vi "Main.vi"(11 "Module Admin":refnum<class "Delacor_lib_QMH_Cloneable Module Admin.lvclass">) -> ()   [LabVIEW 2023, in "EL72xx_DMC_ServoAxis.lvlib"]
doc: "This template is based off of the Queued Message Handler design pattern and the Queued Message Handler project template that ships with LabVIEW.\n\nThe main difference is that the queue is private to this module and communication between modules is performed via Broadcast and Request events.\n\nRequest events are wrapped in public API methods and are handled in the Event Handling Loop (EHL) of this VI. Any module can register for Broadcast events sent by this module. The EHL generates messages based on user interface actions.\n\nThe Message Handling Loop (MHL) processes messages generated by the EHL, or by other messages. The messages are string values, so new messages can be added easily to the Message Cases case structure in the MHL. Each message cluster can also provide an optional value for Message Data, which is a variant that can be converted to whatever message-specific data is required.\n_____\nBased on DQMH Project Template 7.0.1.1316."
uses:
  EL72xx_DMC_ServoAxis.lvlib
  <vilib>/Delacor/Delacor QMH/Libraries/Cloneable Module Admin_class/Delacor_lib_QMH_Cloneable Module Admin.lvclass
  C:/Program Files/National Instruments/LabVIEW 2023/vi.lib/Delacor/Delacor QMH/Libraries/Module Admin_class/Delacor_lib_QMH_Module Admin.lvclass
  Module Data--cluster.ctl
  <vilib>/Delacor/Delacor QMH/Libraries/Message Queue_class/Delacor_lib_QMH_Message Queue.lvclass/Delacor_lib_QMH_Message Queue.ctl
  <vilib>/Delacor/Delacor QMH/Libraries/Cloneable Module Admin_class/Delacor_lib_QMH_Cloneable Module Admin.lvclass/Delacor_lib_QMH_Cloneable Module Admin.ctl
  Stop Argument--cluster.ctl
  <vilib>/Delacor/Delacor QMH/Libraries/Module Admin_class/Delacor_lib_QMH_Module Admin.lvclass/Delacor_lib_QMH_Module Admin.ctl
  Enable_Drive Argument--cluster.ctl
  <vilib>/Utility/miscctls.llb/LVPointTypeDef.ctl
  <vilib>/Delacor/Delacor QMH/Libraries/Message Queue_class/Delacor_lib_QMH_Enqueue Message (Single).vi
  <vilib>/Delacor/Delacor QMH/Libraries/Cloneable Module Admin_class/Delacor_lib_QMH_Get Module ID.vi
  <vilib>/Delacor/Delacor QMH/Libraries/Module Admin_class/Delacor_lib_QMH_Get External Launch.vi
  <vilib>/Delacor/Delacor QMH/Libraries/Message Queue_class/Delacor_lib_QMH_Message Queue.lvclass
  ConnectToDrive Argument--cluster.ctl
  DisconnectFromDrive Argument--cluster.ctl
  DisableDrive Argument--cluster.ctl
  <userlib>/Beckhoff-LabVIEW-Interface/_DependsOn/Base/TypeResolver/Set TypeResolver.vi
  <userlib>/Beckhoff-LabVIEW-Interface/_DependsOn/Base/Write/Write Sync.vi
panel:
  out "error out":errorcluster
  out "Status":string
  in  "Simulate EHL Error":bool
  in  "Simulate MHL Error":bool
  # "Other processes communicate with this Module via its Public API (wrappers for its Request Events).\n\nThis Module communicates with other processes via its Broadcast Events.\nAny process that wants to receive these messages can register for this module's Broadcast events."
  # "This template is for the DQMH framework. See the block diagram for more information on how to use this template."
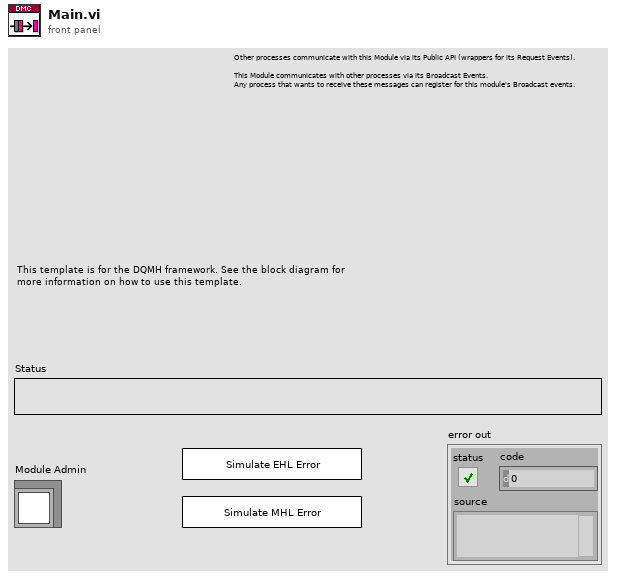
[diagram p1: front panel]
types:
  T1 = typedef "EL72xx_DMC_ServoAxis.lvlib/Request Events--cluster.ctl" = cluster{"Stop Module":refnum<user-event>, "Show Panel":refnum<user-event>, "Hide Panel":refnum<user-event>, "Show Diagram":refnum<user-event>, "Get Module Execution Status":refnum<user-event>, "Enable_Drive":refnum<user-event>, "ConnectToDrive":refnum<user-event>, "DisconnectFromDrive":refnum<user-event>, "DisableDrive":refnum<user-event>}
  T2 = typedef "EL72xx_DMC_ServoAxis.lvlib/Module Data--cluster.ctl" = cluster{"Status":string}
  T3 = enum32{"invalid lock state", "Not Locked", "Locked (No Password)", "Password-protected"}
  T4 = typedef "EL72xx_DMC_ServoAxis.lvlib/Stop Argument--cluster.ctl" = cluster{"Module ID":i32, "Origin":string, "Exit via Stop Module Req?":bool, "Wait for Module to stop?":bool}
  T5 = typedef "EL72xx_DMC_ServoAxis.lvlib/Enable_Drive Argument--cluster.ctl" = cluster{"Module ID":i32, "Enable":bool}
  T6 = typedef "EL72xx_DMC_ServoAxis.lvlib/ConnectToDrive Argument--cluster.ctl" = cluster{"Module ID":i32, "Path":path}
  T7 = typedef "EL72xx_DMC_ServoAxis.lvlib/DisconnectFromDrive Argument--cluster.ctl" = cluster{"Module ID":i32, "Boolean":bool}
  T8 = typedef "EL72xx_DMC_ServoAxis.lvlib/DisableDrive Argument--cluster.ctl" = cluster{"Module ID":i32, "Disable":bool}
  T9 = typedef "LVPointTypeDef.ctl" = cluster{"Horizontal":i16, "Vertical":i16}
  T10 = enum32{"Invalid", "Standard", "Closed", "Hidden", "Minimized", "Maximized"}
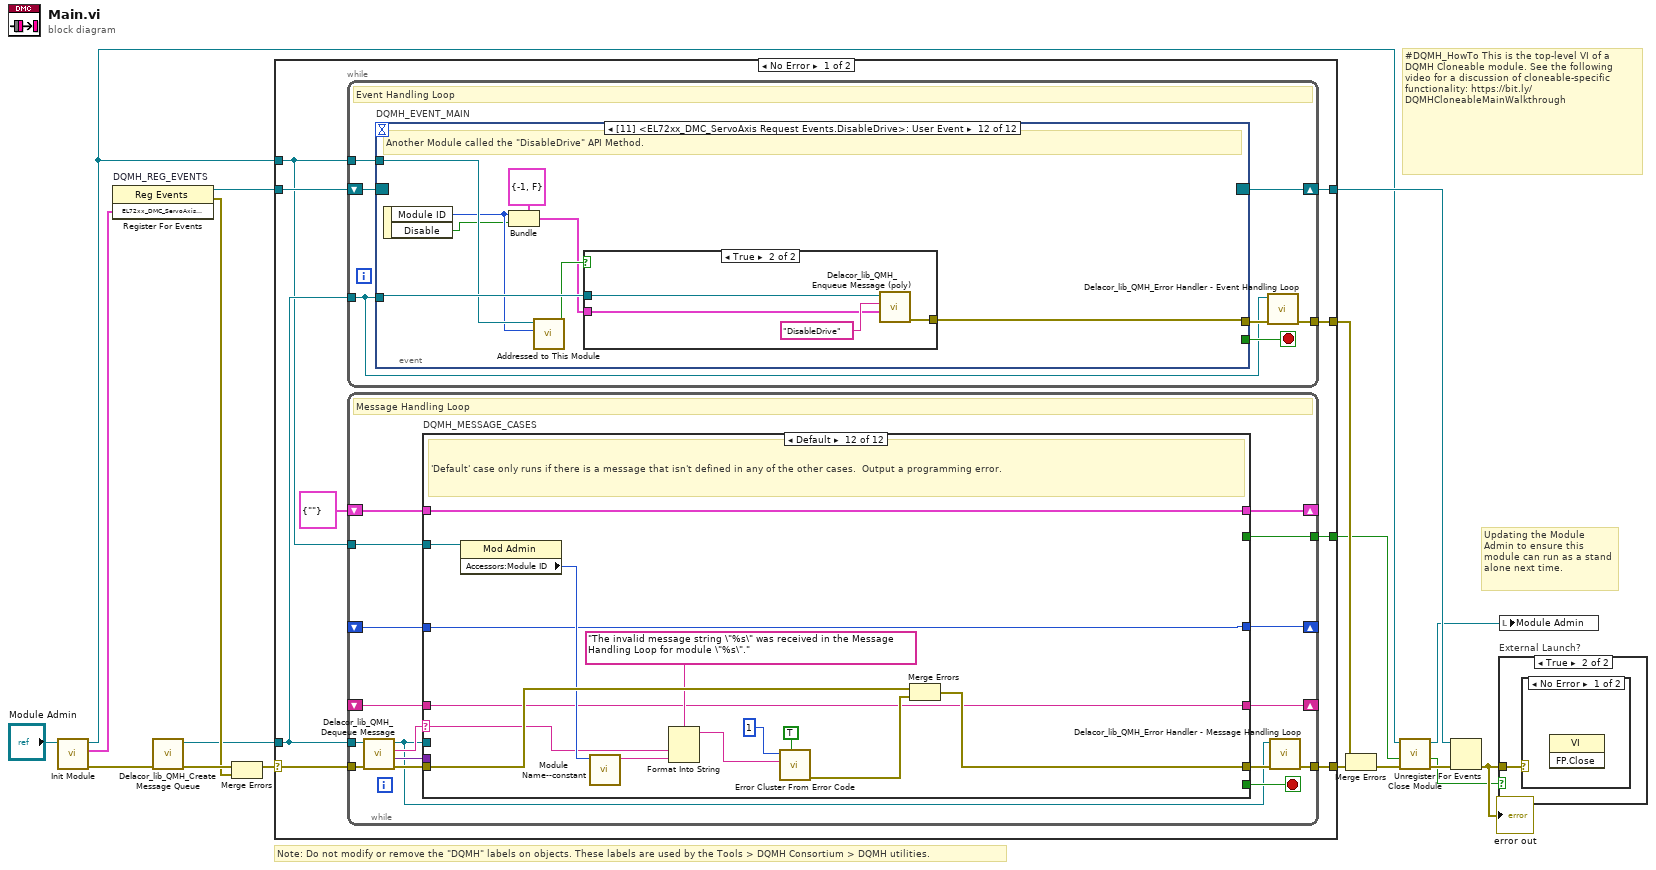
[diagram p0: block diagram]
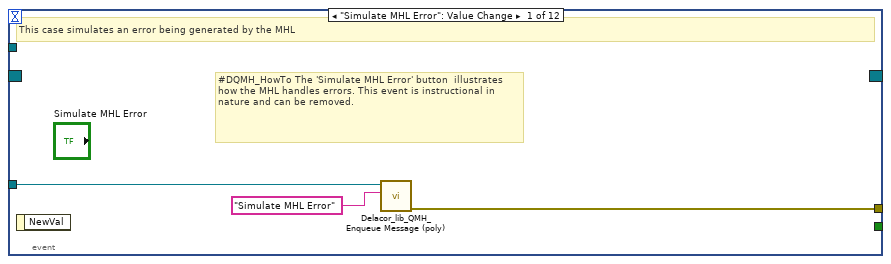
[diagram p2: hidden frame]
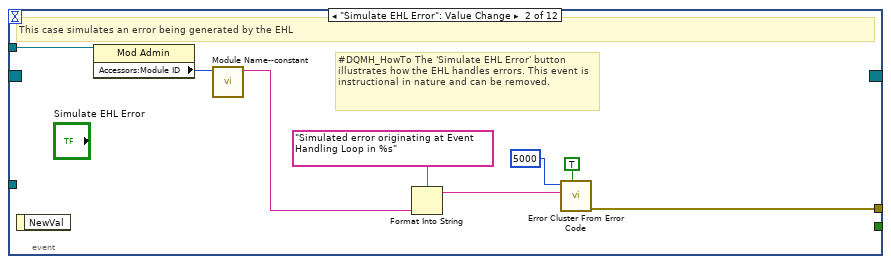
[diagram p3: hidden frame]
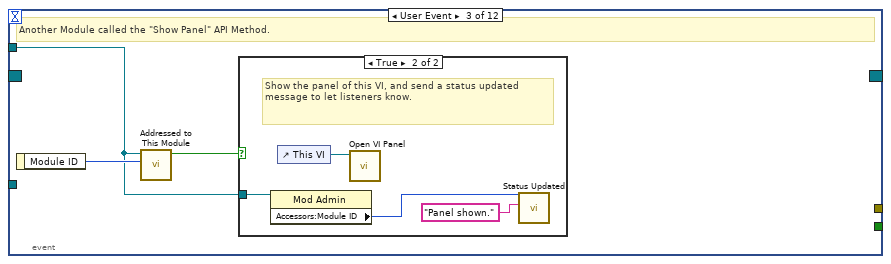
[diagram p4: hidden frame]
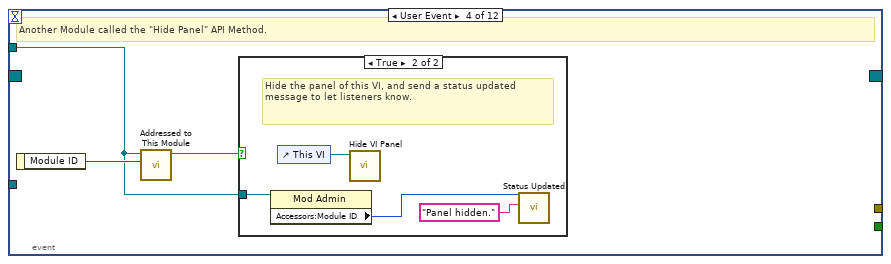
[diagram p6: hidden frame]
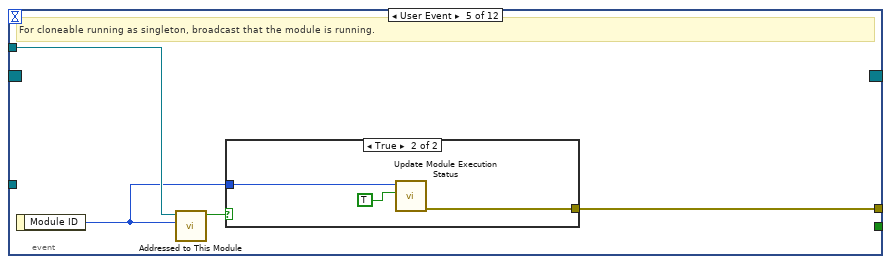
[diagram p8: hidden frame]
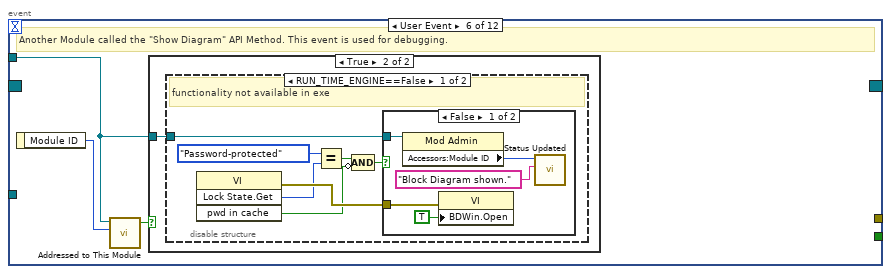
[diagram p10: hidden frame]
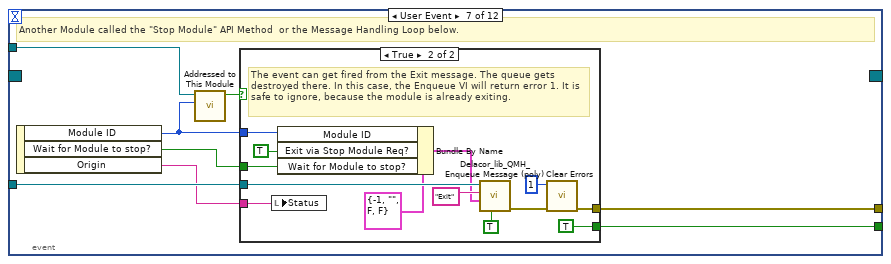
[diagram p14: hidden frame]
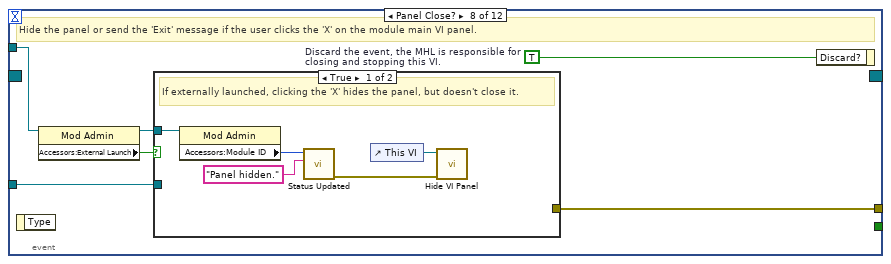
[diagram p16: hidden frame]
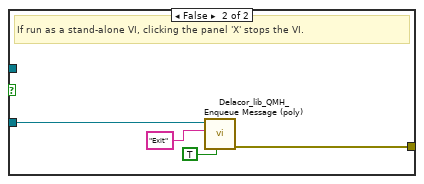
[diagram p17: hidden frame]
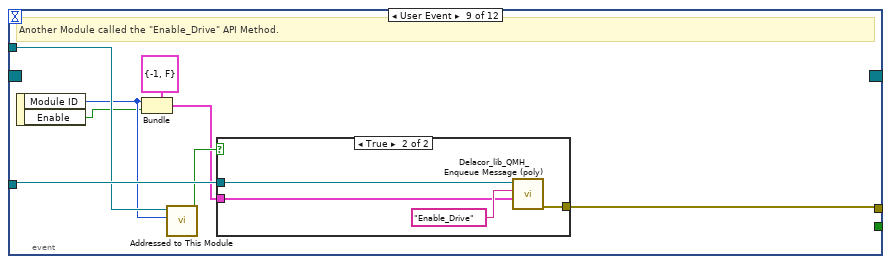
[diagram p18: hidden frame]
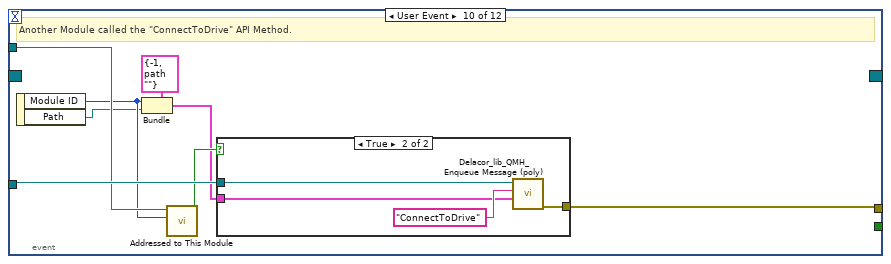
[diagram p20: hidden frame]
diagram:
  # "#DQMH_HowTo This is the top-level VI of a DQMH Cloneable module. See the following video for a discussion of cloneable-specific functionality: https://bit.ly/DQMHCloneableMainWalkthrough"
  # "Note: Do not modify or remove the \"DQMH\" labels on objects. These labels are used by the Tools > DQMH Consortium > DQMH utilities."
  # "Updating the Module Admin to ensure this module can run as a stand alone next time."
  n1 = call "Init Module.vi"("Cloneable Module Admin in"="Module Admin") -> ("error out"=w15:errorcluster, "EL72xx_DMC_ServoAxis Request Events"=w7:T1, "Cloneable Module Admin out"=w4:refnum<class "Delacor_lib_QMH_Cloneable Module Admin.lvclass">)  [unwired: 8 in]
  n2 = register-events "DQMH_REG_EVENTS"(w7) -> (reference out=w8:refnum<event-registration>, error out=w10:errorcluster)  [unwired: 2 in]
  n3 = call <vilib>:"Delacor_lib_QMH_Create Message Queue.vi"("error in"=w15) -> ("error out"=w12:errorcluster, "Message Queue"=w6:refnum<class "Delacor_lib_QMH_Message Queue.lvclass">)  [unwired: 9 in]
  n4 = Merge Errors(w12, w10) -> (w11:errorcluster)
  n5 = case shown="No Error" w11 {
    selector: w11 -> [w25 w348]
    tunnel: [w27 w347] -> w16
    tunnel: [w24 w346] -> w9
    tunnel: w8 -> [w22 w346]
    tunnel: w6 -> [w21 w339]
    tunnel: [w26 _] -> w17
    tunnel: w4 -> [w20 w342]
    tunnel: [w19 _] -> w2
    frame No Error {
      n6 = while {
        tunnel: w21 -> [w28]
        shift-right: [w31] -> w24
        shift-left: w22 -> [w32]
        tunnel: [w33] -> w26
        tunnel: w20 -> [w29]
        stop <- w30 stop-if-true
        # "Event Handling Loop"
        n7 = event "DQMH_EVENT_MAIN" shown="[11] <EL72xx_DMC_ServoAxis Request Events.DisableDrive>: User Event" {
          selector: w32 -> [_ _ _ _ _ _ _ _ _ _ _ _]
          dyn-events: [_ _ _ _ _ _ _ _ _ _ _ _] -> w31
          timeout: _ -> [_ _ _ _ _ _ _ _ _ _ _ _]
          tunnel: [_ _ _ _ _ _ w86 _ _ _ _ _] -> w30
          tunnel: w28 -> [w36 _ _ _ _ _ w89 w106 w126 w138 w150 w162]
          tunnel: [w37 w45 _ _ w63 _ w90 w109 w119 w131 w143 w155] -> w34
          tunnel: w29 -> [_ w44 w46 w53 w61 w67 w88 w107 w124 w136 w148 w160]
          event "Simulate MHL Error": Value Change {
            # "#DQMH_HowTo The 'Simulate MHL Error' button  illustrates how the MHL handles errors. This event is instructional in nature and can be removed."
            # "This case simulates an error being generated by the MHL"
            n8 = event-data() -> ()  [unwired: 1 in, 1 out]
            n9 = call-poly <vilib>:"Delacor_lib_QMH_Enqueue Message (poly).vi"("Message"="Simulate MHL Error", "Message Queue in"=w36) -> ("error out"=w37:errorcluster)  [unwired: 8 in, 1 out]
          }
          event "Simulate EHL Error": Value Change {
            # "#DQMH_HowTo The 'Simulate EHL Error' button  illustrates how the EHL handles errors. This event is instructional in nature and can be removed."
            # "This case simulates an error being generated by the EHL"
            n10 = event-data() -> ()  [unwired: 1 in, 1 out]
            n11 = property on="Property Node" class="Mod Admin"(reference=w44) -> ("Accessors:Module ID"=w43:i32)  [unwired: 1 in, 2 out]
            n12 = call "Module Name--constant.vi"("Module ID"=w43) -> ("Module Name"=w38:string)  [unwired: 10 in]
            n13 = Format Into String(format string="Simulated error originating at Event Handling Loop in %s", w38) -> (resulting string=w41:string)  [unwired: 2 in, 1 out]
            n14 = call <vilib>:"Error Cluster From Error Code.vi"("show call chain? (False)"=TRUE, "error message (\"\")"=w41, "error code (0)"=5000) -> ("error out"=w45:errorcluster)  [unwired: 6 in]
          }
          event User Event {
            # "Another Module called the \"Show Panel\" API Method."
            n15 = event-data() -> ("Module ID"=w47:i32)  [unwired: 1 in]
            n16 = call "Addressed to This Module.vi"("Module ID from Argument"=w47, "Module Admin"=w46) -> ("Addressed to this instance?"=w48:bool)  [unwired: 8 in, 1 out]
            n17 = case shown="True" w48 {
              tunnel: w46 -> [_ w50]
              frame False {
              }
              frame True {
                # "Show the panel of this VI, and send a status updated message to let listeners know."
                n18 = property on="Property Node" class="Mod Admin"(reference=w50) -> ("Accessors:Module ID"=w49:i32)  [unwired: 1 in, 2 out]
                n19 = control-ref of="This VI"() -> (w52:refnum<vi>)
                n20 = call "Open VI Panel.vi"("VI"=w52) -> ()  [unwired: 10 in, 1 out]
                n21 = call "Status Updated.vi"("Status"="Panel shown." ("format string"), "Module ID"=w49) -> ()  [unwired: 9 in, 1 out]
              }
            }
          }
          event User Event {
            # "Another Module called the \"Hide Panel\" API Method."
            n22 = event-data() -> ("Module ID"=w54:i32)  [unwired: 1 in]
            n23 = call "Addressed to This Module.vi"("Module ID from Argument"=w54, "Module Admin"=w53) -> ("Addressed to this instance?"=w55:bool)  [unwired: 8 in, 1 out]
            n24 = case shown="True" w55 {
              tunnel: w53 -> [_ w57]
              frame False {
              }
              frame True {
                # "Hide the panel of this VI, and send a status updated message to let listeners know."
                n25 = property on="Property Node" class="Mod Admin"(reference=w57) -> ("Accessors:Module ID"=w56:i32)  [unwired: 1 in, 2 out]
                n26 = control-ref of="This VI"() -> (w59:refnum<vi>)
                n27 = call "Hide VI Panel.vi"("VI"=w59) -> ()  [unwired: 10 in, 1 out]
                n28 = call "Status Updated.vi"("Status"="Panel hidden." ("format string"), "Module ID"=w56) -> ()  [unwired: 9 in, 1 out]
              }
            }
          }
          event User Event {
            # "For cloneable running as singleton, broadcast that the module is running."
            n29 = event-data() -> ("Module ID"=w60:i32)  [unwired: 1 in]
            n30 = call "Addressed to This Module.vi"("Module ID from Argument"=w60, "Module Admin"=w61) -> ("Addressed to this instance?"=w62:bool)  [unwired: 8 in, 1 out]
            n31 = case shown="True" w62 {
              tunnel: [_ w66] -> w63
              tunnel: w60 -> [_ w65]
              frame False {
              }
              frame True {
                n32 = call "Update Module Execution Status.vi"("Running?"=TRUE, "Module ID"=w65) -> ("error out"=w66:errorcluster)  [unwired: 9 in]
              }
            }
          }
          event User Event {
            # "Another Module called the \"Show Diagram\" API Method. This event is used for debugging."
            n33 = event-data() -> ("Module ID"=w68:i32)  [unwired: 1 in]
            n34 = call "Addressed to This Module.vi"("Module ID from Argument"=w68, "Module Admin"=w67) -> ("Addressed to this instance?"=w69:bool)  [unwired: 8 in, 1 out]
            n35 = case shown="True" w69 {
              tunnel: w67 -> [_ w70]
              frame False {
              }
              frame True {
                n36 = disable-structure shown="RUN_TIME_ENGINE==False" {
                  disable-tunnel: w70 -> [w71 _]
                  frame condition #0 (active) {
                    # "functionality not available in exe"
                    n37 = invoke on="Invoke Node" class="VI" method="Lock State.Get"() -> (error out=w77:errorcluster, "Get Lock State"=w76:T3, "pwd in cache"=w73:bool)  [unwired: 4 in, 1 out]
                    n38 = Equal?(x=T3."Password-protected", y=w76) -> (x = y?=w74:bool)
                    n39 = Compound Arithmetic op=AND(w74, invert w73) -> (w72:bool)
                    n40 = case shown="False" w72 {
                      tunnel: w77 -> [w82 _]
                      tunnel: w71 -> [w79 _]
                      frame False {
                        n41 = property on="Property Node" class="Mod Admin"(reference=w79) -> ("Accessors:Module ID"=w78:i32)  [unwired: 1 in, 2 out]
                        n42 = property on="Property Node" class="VI"(error in=w82, "BDWin.Open"=TRUE ("Block Diagram Window:Open")) -> ()  [unwired: 1 in, 2 out]
                        n43 = call "Status Updated.vi"("Status"="Block Diagram shown." ("format string"), "Module ID"=w78) -> ()  [unwired: 9 in, 1 out]
                      }
                      frame True {
                        # "Password-protected VI, and the password is not in the cache. Do not show the diagram."
                      }
                    }
                  }
                  frame condition #1 {
                  }
                }
              }
            }
          }
          event User Event {
            # "Another Module called the \"Stop Module\" API Method  or the Message Handling Loop below."
            n44 = event-data() -> ("Module ID"=w84:i32, "Wait for Module to stop?"=w85:bool, "Origin"=w83:string)  [unwired: 1 in]
            n45 = call "Addressed to This Module.vi"("Module ID from Argument"=w84, "Module Admin"=w88) -> ("Addressed to this instance?"=w87:bool)  [unwired: 8 in, 1 out]
            n46 = case shown="True" w87 {
              tunnel: [_ w102] -> w90
              tunnel: w89 -> [_ w98]
              tunnel: [_ TRUE] -> w86
              tunnel: w85 -> [_ w93]
              tunnel: w84 -> [_ w95]
              tunnel: w83 -> [_ w91]
              frame False {
              }
              frame True {
                # "The event can get fired from the Exit message. The queue gets destroyed there. In this case, the Enqueue VI will return error 1. It is safe to ignore, because the module is already exiting."
                n47 = local write "Status"(w91) -> ()
                n48 = Bundle By Name(cluster=T4 {"Module ID"=-1, "Origin"="", "Exit via Stop Module Req?"=FALSE, "Wait for Module to stop?"=FALSE} ("Stop Argument"), "Module ID"=w95, "Exit via Stop Module Req?"=TRUE, "Wait for Module to stop?"=w93) -> (w92:T4)
                n49 = call-poly <vilib>:"Delacor_lib_QMH_Enqueue Message (poly).vi"("Priority Message? (F)"=TRUE, "Message Data"=w92, "Message"="Exit", "Message Queue in"=w98) -> ("error out"=w103:errorcluster)  [unwired: 6 in, 1 out]
                n50 = call <vilib>:"Clear Errors.vi"("error in (no error)"=w103, "specific error code to clear (0: all)"=1) -> ("error out"=w102:errorcluster)  [unwired: 4 in, 1 out]
              }
            }
          }
          event Panel Close? {
            w108 = TRUE  # Discard the event, the MHL is responsible for closing and stopping this VI.
            # "Hide the panel or send the 'Exit' message if the user clicks the 'X' on the module main VI panel."
            n51 = event-data() -> ()  [unwired: 1 in, 1 out]
            n52 = property on="Property Node" class="Mod Admin"(reference=w107) -> (reference out=w104:refnum<class "Delacor_lib_QMH_Cloneable Module Admin.lvclass">, "Accessors:External Launch"=w105:bool)  [unwired: 1 in, 1 out]
            n53 = case shown="True" w105 {
              tunnel: w106 -> [_ w117]
              tunnel: [_ w118] -> w109
              tunnel: w104 -> [w112 _]
              frame True {
                # "If externally launched, clicking the 'X' hides the panel, but doesn't close it."
                n54 = property on="Property Node" class="Mod Admin"(reference=w112) -> ("Accessors:Module ID"=w111:i32)  [unwired: 1 in, 2 out]
                n55 = call "Status Updated.vi"("Status"="Panel hidden." ("format string"), "Module ID"=w111) -> ("error out"=w110:errorcluster)  [unwired: 9 in]
                n56 = control-ref of="This VI"() -> (w114:refnum<vi>)
                n57 = call "Hide VI Panel.vi"("error in"=w110, "VI"=w114) -> ()  [unwired: 9 in, 1 out]
              }
              frame False {
                # "If run as a stand-alone VI, clicking the panel 'X' stops the VI."
                n58 = call-poly <vilib>:"Delacor_lib_QMH_Enqueue Message (poly).vi"("Priority Message? (F)"=TRUE, "Message"="Exit", "Message Queue in"=w117) -> ("error out"=w118:errorcluster)  [unwired: 7 in, 1 out]
              }
            }
            n59 = event-data ("Event Filter Node")("Discard?"=w108) -> ()  [unwired: 1 in, 1 out]
          }
          event User Event {
            # "Another Module called the \"Enable_Drive\" API Method."
            n60 = event-data() -> ("Module ID"=w121:i32, "Enable"=w120:bool)  [unwired: 1 in]
            n61 = Bundle(cluster=T5 {"Module ID"=-1, "Enable"=FALSE} ("Enable_Drive Argument"), "Module ID"=w121, "Enable"=w120) -> (w122:T5)
            n62 = call "Addressed to This Module.vi"("Module ID from Argument"=w121, "Module Admin"=w124) -> ("Addressed to this instance?"=w125:bool)  [unwired: 8 in, 1 out]
            n63 = case shown="True" w125 {
              tunnel: w126 -> [_ w130]
              tunnel: w122 -> [_ w128]
              tunnel: [_ w127] -> w119
              frame False {
              }
              frame True {
                n64 = call-poly <vilib>:"Delacor_lib_QMH_Enqueue Message (poly).vi"("Message Data"=w128, "Message"="Enable_Drive", "Message Queue in"=w130) -> ("error out"=w127:errorcluster)  [unwired: 7 in, 1 out]
              }
            }
          }
          event User Event {
            # "Another Module called the \"ConnectToDrive\" API Method."
            n65 = event-data() -> ("Module ID"=w133:i32, "Path"=w132:path)  [unwired: 1 in]
            n66 = Bundle(cluster=T6 {"Module ID"=-1, "Path"=path ""} ("ConnectToDrive Argument"), "Module ID"=w133, "Path"=w132) -> (w134:T6)
            n67 = call "Addressed to This Module.vi"("Module ID from Argument"=w133, "Module Admin"=w136) -> ("Addressed to this instance?"=w137:bool)  [unwired: 8 in, 1 out]
            n68 = case shown="True" w137 {
              tunnel: w138 -> [_ w142]
              tunnel: w134 -> [_ w140]
              tunnel: [_ w139] -> w131
              frame False {
              }
              frame True {
                n69 = call-poly <vilib>:"Delacor_lib_QMH_Enqueue Message (poly).vi"("Message Data"=w140, "Message"="ConnectToDrive", "Message Queue in"=w142) -> ("error out"=w139:errorcluster)  [unwired: 7 in, 1 out]
              }
            }
          }
          event User Event {
            # "Another Module called the \"DisconnectFromDrive\" API Method."
            n70 = event-data() -> ("Module ID"=w145:i32, "Boolean"=w144:bool)  [unwired: 1 in]
            n71 = Bundle(cluster=T7 {"Module ID"=-1, "Boolean"=FALSE} ("DisconnectFromDrive Argument"), "Module ID"=w145, "Boolean"=w144) -> (w146:T7)
            n72 = call "Addressed to This Module.vi"("Module ID from Argument"=w145, "Module Admin"=w148) -> ("Addressed to this instance?"=w149:bool)  [unwired: 8 in, 1 out]
            n73 = case shown="True" w149 {
              tunnel: w150 -> [_ w154]
              tunnel: w146 -> [_ w152]
              tunnel: [_ w151] -> w143
              frame False {
              }
              frame True {
                n74 = call-poly <vilib>:"Delacor_lib_QMH_Enqueue Message (poly).vi"("Message Data"=w152, "Message"="DisconnectFromDrive", "Message Queue in"=w154) -> ("error out"=w151:errorcluster)  [unwired: 7 in, 1 out]
              }
            }
          }
          event User Event {
            # "Another Module called the \"DisableDrive\" API Method."
            n75 = event-data() -> ("Module ID"=w157:i32, "Disable"=w156:bool)  [unwired: 1 in]
            n76 = Bundle(cluster=T8 {"Module ID"=-1, "Disable"=FALSE} ("DisableDrive Argument"), "Module ID"=w157, "Disable"=w156) -> (w158:T8)
            n77 = call "Addressed to This Module.vi"("Module ID from Argument"=w157, "Module Admin"=w160) -> ("Addressed to this instance?"=w161:bool)  [unwired: 8 in, 1 out]
            n78 = case shown="True" w161 {
              tunnel: w162 -> [_ w166]
              tunnel: w158 -> [_ w164]
              tunnel: [_ w163] -> w155
              frame False {
              }
              frame True {
                n79 = call-poly <vilib>:"Delacor_lib_QMH_Enqueue Message (poly).vi"("Message Data"=w164, "Message"="DisableDrive", "Message Queue in"=w166) -> ("error out"=w163:errorcluster)  [unwired: 7 in, 1 out]
              }
            }
          }
        }
        n80 = call-dynamic "Delacor_lib_QMH_Error Handler - Event Handling Loop.vi"("error in"=w34, "Message Queue in"=w28) -> ("dup error in"=w33:errorcluster)  [unwired: 8 in, 1 out]
      }
      n81 = while {
        tunnel: w21 -> [w171]
        shift-right: [w178] -> _
        shift-left: T2 {"Status"=""} ("Data Cluster") -> [w179]
        tunnel: w25 -> [w182]
        tunnel: [w180] -> w27
        tunnel: w20 -> [w173]
        tunnel: [w172] -> w19
        shift-right: [w170] -> _
        shift-left: _ -> [w169]
        shift-right: [w168] -> _
        shift-left: _ -> [w167]
        stop <- w177 stop-if-true
        # "Message Handling Loop"
        n82 = call-dynamic "Delacor_lib_QMH_Dequeue Message.vi"("error in"=w182, "Message Queue in"=w171) -> ("error out"=w181:errorcluster, "Message Data"=w175:variant, "Message"=w176:string, "Message Queue out"=w174:refnum<class "Delacor_lib_QMH_Message Queue.lvclass">)  [unwired: 6 in]
        n83 = case "DQMH_MESSAGE_CASES" shown="Default" w176 {
          selector: w176 -> [_ _ _ _ _ _ _ _ _ _ _ w328]
          tunnel: w174 -> [_ _ _ _ _ _ _ _ w277 _ w318 _]
          tunnel: w181 -> [w204 w210 w225 w238 w248 w263 w268 w272 w286 w305 w324 w337]
          tunnel: [w202 w210 w215 w230 w241 w251 w267 w272 w282 w304 w319 w338] -> w183
          tunnel: w179 -> [w195 w209 w224 w237 w247 w262 w266 w271 w281 w302 w317 w335]
          tunnel: [w194 w209 w224 w237 w247 w262 w266 w271 w281 w302 w317 w335] -> w178
          tunnel: [_ _ _ _ _ _ _ _ _ _ w316 _] -> w177
          tunnel: w175 -> [_ _ w223 w236 w246 w261 _ _ w280 _ w314 _]
          tunnel: w173 -> [w189 _ _ _ _ _ _ _ w279 w300 w309 w334]
          tunnel: [_ _ _ _ _ _ _ _ _ _ w312 _] -> w172
          tunnel: [w185 w208 w217 w229 u32 0 ("Handle") w250 w265 w270 w274 w294 w307 w326] -> w170
          tunnel: w169 -> [w185 w208 w220 _ w243 w255 w265 w270 w274 w294 w307 w326]
          tunnel: [w184 w207 w211 w226 "" ("ReadGrpSymbols") w249 w264 w269 w273 w293 w306 w325] -> w168
          tunnel: w167 -> [w184 w207 w212 _ _ w253 w264 w269 w273 w293 w306 w325]
          frame "Initialize" {
            w186 = "Initial Message" ("Initial Message")
            # "#CodeNeeded - Initialize the appearance of the front panel."
            # "#CodeNeeded - Initialize your state data here."
            # "Initialize - Any operation that needs to be done before the module can receive messages. Synchronize Caller Events.vi will inform Start Module.vi that the module has launched and is ready to receive messages. Module Did Init.vi will broadcast that the module initialized."
            n84 = call "Synchronize Caller Events.vi"("error in"=w204, "Module Admin"=w189) -> ("error out"=w203:errorcluster, "Module Admin out"=w188:refnum<class "Delacor_lib_QMH_Cloneable Module Admin.lvclass">)  [unwired: 8 in]
            n85 = property on="Property Node" class="Mod Admin"(reference=w188) -> ("Accessors:Module ID"=w191:i32, "Accessors:External Launch"=w190:bool)  [unwired: 1 in, 2 out]
            n86 = call "Module Name--constant.vi"("Module ID"=w191) -> ("Module Name"=w199:string)  [unwired: 10 in]
            n87 = property on="Property Node" class="VI"("Front Panel.Title"=w199) -> (reference out=w201:refnum<vi>, error out=w206:errorcluster)  [unwired: 2 in]
            n88 = Select(t=T10."Hidden" ("State"), s=w190, f=T10."Standard" ("State")) -> (s? t:f=w196:T10)
            n89 = invoke on="Invoke Node" class="VI" method="FP.Open"(reference=w201, error in=w206, "State"=w196) -> (reference out=w200:refnum<vi>, error out=w205:errorcluster)  [unwired: 2 in, 3 out]
            n90 = call "Module Name--constant.vi"("Module ID"=w191) -> ("Module Name"=w192:string)  [unwired: 10 in]
            n91 = Bundle By Name(cluster=w195, "Status"=w186) -> (w194:T2)
            n92 = invoke on="Invoke Node" class="VI" method="FP.Center"(reference=w200, error in=w205) -> ()  [unwired: 1 in, 3 out]
            n93 = property on="Pane" class="Pane"("Origin"=T9 {"Horizontal"=0, "Vertical"=0}) -> ()  [unwired: 2 in, 2 out]
            n94 = call "Module Did Init.vi"("error in"=w203, "Initialized?"=TRUE, "Origin"=w192, "Module ID"=w191) -> ("error out"=w202:errorcluster)  [unwired: 7 in]
            "Status" <- w186
          }
          frame "---Module Specific---" {
            # "Separator -- The following cases handle messages specific to this Module."
          }
          frame "Enable_Drive" {
            # "Enable the EL72xx drive unit"
            n95 = Variant To Data(error in=w225, type=T5 {"Module ID"=-1, "Enable"=FALSE} ("Enable_Drive Argument"), Variant=w223) -> (data=w221:T5, error out=w219:errorcluster)
            n96 = Unbundle By Name(w221) -> ("Enable"=w214:bool)  [unwired: 1 out]
            n97 = call-poly <userlib>:"TypeResolver.vi"("Handle"=w220, "SymbolName"=w212, "WData"=w214, "error in"=w219) -> ("Handle"=w218:u32, "ADSWData"=w213:variant, "error out"=w216:errorcluster)  [unwired: 8 in, 1 out]
            n98 = call-poly <userlib>:"ADS Write.vi"("Handle"=w218, "SymbolName"=w212, "Ads Write Data"=w213, "error in (no error)"=w216) -> ("Handle"=w217:u32, "SymbolName"=w211:string, "error out"=w215:errorcluster)  [unwired: 8 in, 1 out]
          }
          frame "ConnectToDrive" {
            w227 = 0 ("index")
            # "Initiate connection to drive"
            n99 = Variant To Data(error in=w238, type=T6 {"Module ID"=-1, "Path"=path ""} ("ConnectToDrive Argument"), Variant=w236) -> (data=w234:T6, error out=w231:errorcluster)
            n100 = Unbundle By Name(w234) -> ("Path"=w233:path)  [unwired: 1 out]
            n101 = Path To String(path=w233) -> (string=w232:string)
            n102 = call <userlib>:"Init.vi"("XMLDescription"=w232, "error in (no error)"=w231) -> ("Handle"=w229:u32, "ReadGrpSymbols"=w228:string[], "error out"=w230:errorcluster)  [unwired: 9 in, 2 out]
            n103 = Index Array(array=w228, index=w227) -> (element=w226:string)
            n104 = Index Array(array=w228, index=w227) -> ()  [unwired: 1 out]
          }
          frame "DisconnectFromDrive" {
            # "close the connection to the drive unit"
            n105 = Variant To Data(error in=w248, type=T7 {"Module ID"=-1, "Boolean"=FALSE} ("DisconnectFromDrive Argument"), Variant=w246) -> (data=w244:T7, error out=w242:errorcluster)
            n106 = Unbundle By Name(w244) -> ()  [unwired: 2 out]
            n107 = call <userlib>:"Release.vi"("Handle"=w243, "error in (no error)"=w242) -> ("error out"=w241:errorcluster)  [unwired: 13 in]
          }
          frame "DisableDrive" {
            # "Disable the drive unit"
            n108 = Variant To Data(error in=w263, type=T8 {"Module ID"=-1, "Disable"=FALSE} ("DisableDrive Argument"), Variant=w261) -> (data=w259:T8, error out=w252:errorcluster)
            n109 = Unbundle By Name(w259) -> ("Disable"=w254:bool)  [unwired: 1 out]
            n110 = call-poly <userlib>:"TypeResolver.vi"("Handle"=w255, "SymbolName"=w253, "WData"=w254, "error in"=w252) -> ("Handle"=w256:u32, "ADSWData"=w258:variant, "error out"=w257:errorcluster)  [unwired: 8 in, 1 out]
            n111 = call-poly <userlib>:"ADS Write.vi"("Handle"=w256, "SymbolName"=w253, "Ads Write Data"=w258, "error in (no error)"=w257) -> ("Handle"=w250:u32, "SymbolName"=w249:string, "error out"=w251:errorcluster)  [unwired: 8 in, 1 out]
          }
          frame "---Copy This Frame---" {
            # "Duplicate this frame when creating new messages.  Change this comment in the duplicated frame to describe this message."
            n112 = Merge Errors(w268) -> (w267:errorcluster)
          }
          frame "---Exit and Error Handling---" {
            # "Separator - the following cases handle errors and exit messages."
          }
          frame "Error" {
            # "#CodeRecommended - If the module is running in standalone mode (External Launch = FALSE), this code will pop up an error dialog and call the 'Exit' message if an error occurs. Add more fine-grained error management here."
            # "Error - Check the error message data and respond accordingly. This message is sent by the \"Error Handler\" VIs at the end of each loop in this application."
            n113 = property on="Property Node" class="Mod Admin"(reference=w279) -> ("Accessors:External Launch"=w278:bool, "Accessors:Module ID"=w276:i32)  [unwired: 1 in, 2 out]
            n114 = Variant To Data(error in=w286, type=errorcluster {"status"=FALSE, "code"=0, "source"=""} ("error constant"), Variant=w280) -> (data=w275:errorcluster, error out=w284:errorcluster)
            n115 = local write "error out"(w275) -> ()
            n116 = call "Error Reported.vi"("Error"=w275, "Module ID"=w276) -> ()  [unwired: 9 in, 1 out]
            n117 = case shown="False" w278 {
              tunnel: [w291 _] -> w283
              tunnel: w277 -> [w289 _]
              tunnel: w275 -> [w290 _]
              frame False {
                n118 = disable-structure shown="Default" {
                  disable-tunnel: w290 -> [w292 _]
                  frame condition #0 (active) {
                    # "If the module is running standalone, then pop up an error dialog and call the \"Exit\" message."
                    n119 = call <vilib>:"Simple Error Handler.vi"("error in (no error)"=w292) -> ()  [unwired: 4 in, 5 out]
                  }
                  frame condition #1 {
                    # "To prevent the Simple Error Handler VI from being loaded (e.g. when deploying to a Real-Time target), add the Conditional Disable Symbol \"DQMH_Disable_SEH\" to your project and set it to TRUE."
                  }
                }
                n120 = call-poly <vilib>:"Delacor_lib_QMH_Enqueue Message (poly).vi"("Priority Message? (F)"=TRUE, "Message"="Exit", "Message Queue in"=w289) -> ("error out"=w291:errorcluster)  [unwired: 7 in, 1 out]
              }
              frame True {
                # "If the module was launched externally, calling the Error Reported broadcast VI is the only action performed by the \"Error\" message. The module's caller can then process the error appropriately."
              }
            }
            n121 = Merge Errors(w284, w283) -> (w282:errorcluster)
          }
          frame "Simulate MHL Error" {
            # "#DQMH_HowTo The 'Simulate MHL Error' button  illustrates how the MHL handles errors. This event is instructional in nature and can be removed."
            # "Simulate an error occurring at the MHL"
            n122 = property on="Property Node" class="Mod Admin"(reference=w300) -> ("Accessors:Module ID"=w301:i32)  [unwired: 1 in, 2 out]
            n123 = call "Module Name--constant.vi"("Module ID"=w301) -> ("Module Name"=w296:string)  [unwired: 10 in]
            n124 = Format Into String(format string="Simulated error originating at Message Handling Loop in %s", w296) -> (resulting string=w297:string)  [unwired: 2 in, 1 out]
            n125 = call <vilib>:"Error Cluster From Error Code.vi"("show call chain? (False)"=TRUE, "error message (\"\")"=w297, "error code (0)"=5001) -> ("error out"=w303:errorcluster)  [unwired: 6 in]
            n126 = Merge Errors(w305, w303) -> (w304:errorcluster)
          }
          frame "Exit" {
            w315 = 91  # 91: not all Exit messages will have an argument
            w316 = TRUE  # Stop the VI
            # "Release the message queue reference"
            # "#CodeNeeded - Add any required cleanup code here."
            # "Exit - Exit the application."
            n127 = Variant To Data(error in=w324, type=T4 {"Module ID"=-1, "Origin"="", "Exit via Stop Module Req?"=FALSE, "Wait for Module to stop?"=FALSE} ("Stop Argument"), Variant=w314) -> (data=w311:T4, error out=w320:errorcluster)
            n128 = call <vilib>:"Clear Errors.vi"("error in (no error)"=w320, "specific error code to clear (0: all)"=w315) -> ("error out"=w323:errorcluster)  [unwired: 4 in, 1 out]
            n129 = property on="Property Node" class="Mod Admin"(reference=w309) -> ("Accessors:Module ID"=w308:i32)  [unwired: 1 in, 2 out]
            n130 = control-ref of="This VI"() -> (w310:refnum<vi>)
            n131 = call-dynamic "Delacor_lib_QMH_Release Message Queue.vi"("error in"=w323, "Message Queue"=w318) -> ("error out"=w322:errorcluster)  [unwired: 9 in]
            n132 = call "Handle Exit.vi"("Stop Argument"=w311, "Module Admin in"=w309, "VI reference"=w310) -> ("error out"=w321:errorcluster, "Wait for Stop?"=w312:bool)  [unwired: 7 in]
            n133 = Merge Errors(w322, w321) -> (w319:errorcluster)
            n134 = call "Error Reported.vi"("Error"=w319, "Module ID"=w308) -> ()  [unwired: 9 in, 1 out]
          }
          frame Default {
            # "'Default' case only runs if there is a message that isn't defined in any of the other cases.  Output a programming error."
            n135 = property on="Property Node" class="Mod Admin"(reference=w334) -> ("Accessors:Module ID"=w333:i32)  [unwired: 1 in, 2 out]
            n136 = call "Module Name--constant.vi"("Module ID"=w333) -> ("Module Name"=w327:string)  [unwired: 10 in]
            n137 = Format Into String(format string="The invalid message string \"%s\" was received in the Message Handling Loop for module \"%s\".", w328, w327) -> (resulting string=w330:string)  [unwired: 2 in, 1 out]
            n138 = call <vilib>:"Error Cluster From Error Code.vi"("show call chain? (False)"=TRUE, "error message (\"\")"=w330, "error code (0)"=1) -> ("error out"=w336:errorcluster)  [unwired: 6 in]
            n139 = Merge Errors(w337, w336) -> (w338:errorcluster)
          }
        }
        n140 = call-dynamic "Delacor_lib_QMH_Error Handler - Message Handling Loop.vi"("error in"=w183, "Message Queue in"=w174) -> ("dup error in"=w180:errorcluster)  [unwired: 8 in, 1 out]
      }
    }
    frame Error {
      n141 = call "Synchronize Caller Events.vi"("Module Admin"=w342) -> ("Module Admin out"=w341:refnum<class "Delacor_lib_QMH_Cloneable Module Admin.lvclass">)  [unwired: 9 in, 1 out]
      n142 = property on="Property Node" class="Mod Admin"(reference=w341) -> ("Accessors:Module ID"=w340:i32)  [unwired: 1 in, 2 out]
      n143 = call-dynamic "Delacor_lib_QMH_Release Message Queue.vi"("error in"=w348, "Message Queue"=w339) -> ("error out"=w347:errorcluster)  [unwired: 9 in]
      n144 = call "Module Name--constant.vi"("Module ID"=w340) -> ("Module Name"=w345:string)  [unwired: 10 in]
      n145 = Format Into String(format string="An error occurred during initialization. %s is no longer running.", w345) -> (resulting string=w343:string)  [unwired: 2 in, 1 out]
      n146 = call "Error Reported.vi"("Additional Information"=w343, "Error"=w347, "Module ID"=w340) -> ()  [unwired: 8 in, 1 out]
    }
  }
  n147 = Merge Errors(w17, w16) -> (w18:errorcluster)
  n148 = call "Close Module.vi"("error in"=w18, "Wait for stop?"=w2, "Module Admin in"=w4) -> ("error out"=w14:errorcluster, "External Launch"=w1:bool, "Module Admin out"=w3:refnum<class "Delacor_lib_QMH_Cloneable Module Admin.lvclass">)  [unwired: 6 in]
  n149 = Unregister For Events(event registration refnum=w9, error in=w14) -> (error out=w13:errorcluster)
  "error out" <- w13
  n150 = case "External Launch?" shown="True" w1 {
    tunnel: w13 -> [_ w349]
    frame False {
    }
    frame True {
      n151 = case shown="No Error" w349 {
        frame No Error {
          n152 = invoke class="VI" method="FP.Close"() -> ()  [unwired: 3 in, 3 out]
        }
        frame Error {
          n153 = invoke class="VI" method="FP.Open"("Activate"=TRUE ("Activate?")) -> ()  [unwired: 4 in, 5 out]
        }
      }
    }
  }
  n154 = local write "Module Admin"(w3) -> ()
